vi "ActionVIOnCompile.vi"(8 "error in":errorcluster, 11 "Device Item Ref in":T1 format="%.0x") -> (0 "error out":errorcluster)   [LabVIEW 2017, in "NI-XNET Monitor System Explorer.lvlib"]
uses:
  NI-XNET Monitor System Explorer.lvlib
  <vilib>/NI Veristand/Custom Device API/Custom Device Item Ref.ctl
  Shared/Compiled.Data.ctl
  Shared/Constants.vi
  <vilib>/NI Veristand/Custom Device Tools/Custom Device Utility Library/NI VeriStand - Search for All Items by GUID.vi
  <vilib>/NI Veristand/Custom Device API/Get Item Property (String).vi
  <vilib>/NI Veristand/Custom Device API/Set Item Property (Variant).vi
  <vilib>/NI VeriStand/Custom Device Tools/Custom Device Utility Library/Custom Device Utility Library.lvlib
  <vilib>/NI Veristand/Custom Device API/Custom Device API.lvlib
  Shared/NI-XNET Monitor Shared.lvlib
  <vilib>/NI/NIVS Inline Async API/_Data Access System Explorer/Data Access System Explorer.lvlib
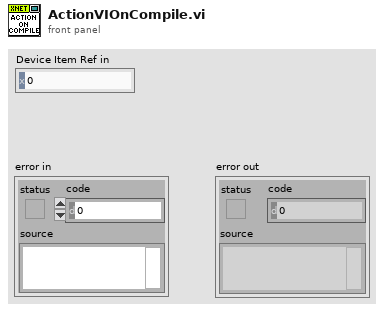
[diagram p1: front panel]
types:
  T1 = typedef "Custom Device API.lvlib/Custom Device Item Ref.ctl" = u64
  T2 = typedef "NI-XNET Monitor Shared.lvlib/Compiled.Data.ctl" = cluster{"CAN":string[], "FlexRay":string[], "LIN":string[], "Async Loop Rate (s)":dbl}
  T3 = enum16{"Output/Write", "Input/Read", "Input/ReadWrite"}
  T4 = cluster{"Name":string, "Type":enum16{"Output/Write", "Input/Read", "Input/ReadWrite"}, "VS Refs":T1[]}
  T5 = typedef "Custom Device API.lvlib/Custom Device Item Info.ctl" = cluster{"Name":string, "Is Channel":bool, "GUID":string, "Is Waveform":bool}
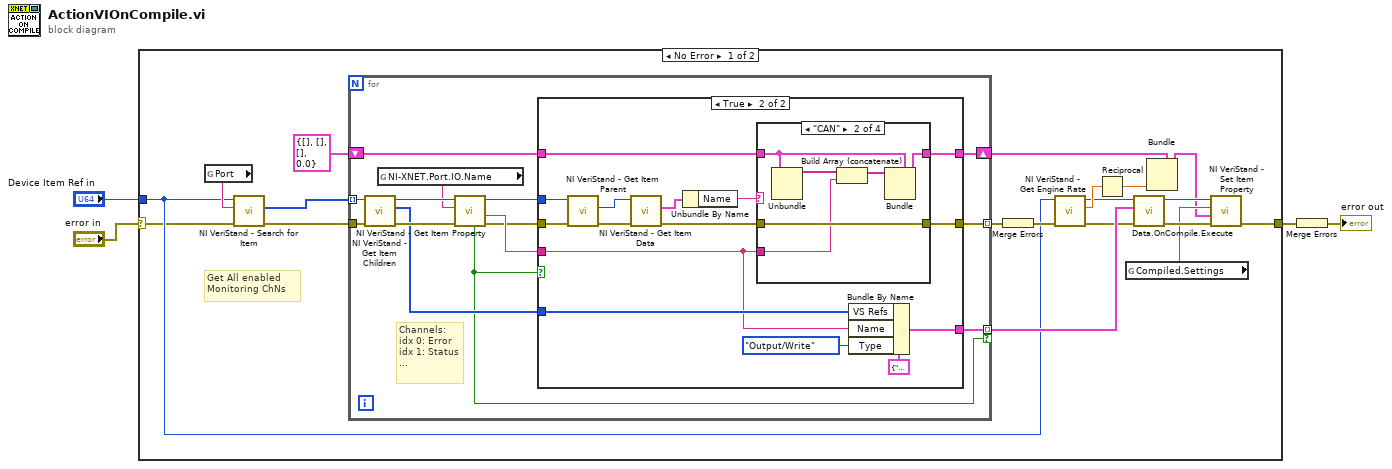
[diagram p0: block diagram]
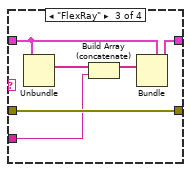
[diagram p4: hidden frame]
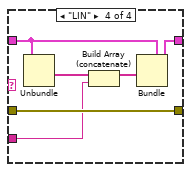
[diagram p5: hidden frame]
diagram:
  n1 = case shown="No Error" "error in" {
    selector: "error in" -> [w7 w75]
    tunnel: [w16 w75] -> w2
    tunnel: "Device Item Ref in" -> [w8 _]
    frame No Error {
      # "Get All enabled\nMonitoring ChNs"
      n2 = global read "Constants.vi" "Port"() -> (w22:string)
      n3 = call-poly <vilib>:"NI VeriStand - Search for Item.vi"("error in"=w7, "Item GUID"=w22, "Section Ref in"=w8) -> ("error out"=w20:errorcluster, "Item Refs"=w21:T1[])  [unwired: 5 in, 2 out]
      n4 = for {
        tunnel: w21 -> [w32] mode=indexing
        tunnel: w20 -> [w37]
        shift-right: [w35] -> w17
        shift-left: T2 {"CAN"=[], "FlexRay"=[], "LIN"=[], "Async Loop Rate (s)"=0.0} -> [w34]
        tunnel: [w33] -> w23 mode=indexing
        tunnel: [w26] -> w19 mode=indexing if=w24
        # "Channels:\nidx 0: Error \nidx 1: Status\n..."
        n5 = call <vilib>:"NI VeriStand - Get Item Children.vi"("error in (no error)"=w37, "Item Ref in"=w32) -> ("error out"=w36:errorcluster, "Child Refs"=w25:T1[], "Item Ref out"=w31:T1)  [unwired: 6 in, 1 out]
        n6 = global read "Constants.vi" "NI-XNET.Port.IO.Name"() -> (w30:string)
        n7 = call-poly <vilib>:"NI VeriStand - Get Item Property.vi"("error in (no error)"=w36, "Property Name"=w30, "Item Ref in"=w31) -> ("error out"=w27:errorcluster, "Value"=w28:string, "Item Ref out"=w29:T1, "Found?"=w24:bool)  [unwired: 5 in]
        n8 = case shown="True" w24 {
          tunnel: w29 -> [_ w51]
          tunnel: w25 -> [_ w42]
          tunnel: [w39 w54] -> w35
          tunnel: w34 -> [w39 w53]
          tunnel: [w38 w52] -> w33
          tunnel: w28 -> [_ w40]
          tunnel: w27 -> [w38 w46]
          tunnel: [_ w43] -> w26
          frame False {
          }
          frame True {
            n9 = call <vilib>:"NI VeriStand - Get Item Parent.vi"("error in (no error)"=w46, "Item Ref in"=w51) -> ("error out"=w48:errorcluster, "Parent Ref"=w49:T1)  [unwired: 6 in, 2 out]
            n10 = call <vilib>:"NI VeriStand - Get Item Data.vi"("error in (no error)"=w48, "Item Ref in"=w49) -> ("error out"=w47:errorcluster, "Item Info"=w50:T5)  [unwired: 6 in, 2 out]
            n11 = Unbundle By Name(w50) -> ("Name"=w45:string)
            n12 = case shown="\"CAN\"" w45 {
              tunnel: w47 -> [w55 w59 w65 w71]
              tunnel: [w56 w62 w68 w73] -> w54
              tunnel: w53 -> [w56 w61 w67 w74]
              tunnel: [w55 w59 w65 w71] -> w52
              tunnel: w40 -> [_ w58 w64 w69]
              frame Default {
              }
              frame "CAN" {
                # "CAN Interface"
                n13 = Unbundle(w61) -> ("CAN"=w60:string[])  [unwired: 3 out]
                n14 = Build Array (concatenate)(w60, w58) -> (w57:string[])
                n15 = Bundle(cluster=w61, "CAN"=w57) -> (w62:T2)  [unwired: 3 in]
              }
              frame "FlexRay" {
                # "FlexRay Interface"
                n16 = Unbundle(w67) -> ("FlexRay"=w66:string[])  [unwired: 3 out]
                n17 = Build Array (concatenate)(w66, w64) -> (w63:string[])
                n18 = Bundle(cluster=w67, "FlexRay"=w63) -> (w68:T2)  [unwired: 3 in]
              }
              frame "LIN" {
                # "LIN Interface"
                n19 = Unbundle(w74) -> ("LIN"=w72:string[])  [unwired: 3 out]
                n20 = Build Array (concatenate)(w72, w69) -> (w70:string[])
                n21 = Bundle(cluster=w74, "LIN"=w70) -> (w73:T2)  [unwired: 3 in]
              }
            }
            n22 = Bundle By Name(cluster=T4 {"Name"="", "Type"=enum."Input/Read", "VS Refs"=[]} ("Group"), "VS Refs"=w42, "Name"=w40, "Type"=T3."Output/Write") -> (w43:T4)
          }
        }
      }
      n23 = Merge Errors(w23) -> (w11:errorcluster)
      n24 = call <vilib>:"NI VeriStand - Get Engine Rate.vi"("error in (no error)"=w11, "Item Ref in"=w8) -> ("error out"=w10:errorcluster, "Rate (Hz)"=w12:dbl, "Item Ref out"=w9:T1)  [unwired: 7 in]
      n25 = Reciprocal(x=w12) -> (1/x=w5:dbl)
      n26 = global read "Constants.vi" "Compiled.Settings"() -> (w13:string)
      n27 = call <vilib>:"Data.OnCompile.Execute.vi"("error in"=w10, "VS Ref Groups"=w19, "Custom Device Ref"=w9) -> ("error out"=w15:errorcluster, "Custom Device Ref"=w18:T1)  [unwired: 7 in]
      n28 = Bundle(cluster=w17, "Async Loop Rate (s)"=w5) -> (w6:T2)  [unwired: 3 in]
      n29 = call-poly <vilib>:"NI VeriStand - Set Item Property.vi"("error in (no error)"=w15, "Value"=w6, "Property Name"=w13, "Item Ref in"=w18) -> ("error out"=w16:errorcluster)  [unwired: 5 in, 2 out]
    }
    frame Error {
    }
  }
  n30 = Merge Errors(w2) -> (→"error out":errorcluster)
